vi "_Set BD Cluster Autosizing Property.vi"(8 "error in (no error)":errorcluster, 10 "type":T1(ring), 11 "SelList[]":refnum<vi>[](array[refnum])) -> (0 "error out":errorcluster, 3 "changed":bool)   [LabVIEW 2020, in "Cluster AutoSizing.lvlib"]
uses:
  Cluster AutoSizing.lvlib
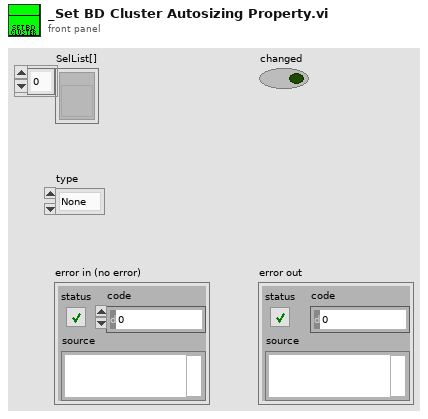
[diagram p1: front panel]
types:
  T1 = enum16{"None", "Size to Fit", "Arrange Horizontally", "Arrange Veritcally"}
  T2 = enum32{"None", "Size to Fit", "Arrange Horizontally", "Arrange Vertically"}
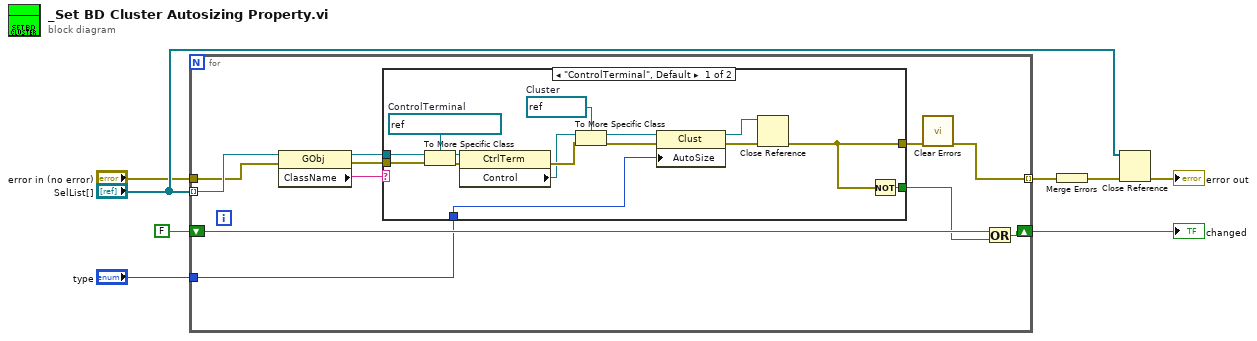
[diagram p0: block diagram]
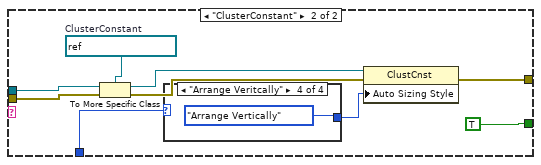
[diagram p2: hidden frame]
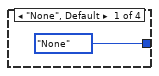
[diagram p3: hidden frame]
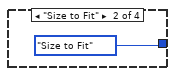
[diagram p4: hidden frame]
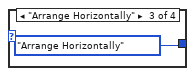
[diagram p5: hidden frame]
diagram:
  n1 = for {
    shift-right: [w18] -> w3
    shift-left: FALSE -> [w19]
    tunnel: "SelList[]" -> [w17] mode=indexing
    tunnel: "error in (no error)" -> [w12]
    tunnel: [w9] -> w4 mode=indexing
    tunnel: "type" -> [w16]
    n2 = property class="GObj"(reference=w17, error in=w12) -> (reference out=w14:refnum<vi>, error out=w13:errorcluster, "ClassName"=w11:string)
    n3 = case shown="\"ControlTerminal\", Default" w11 {
      tunnel: w16 -> [w20 w36]
      tunnel: [w21 w43] -> w15
      tunnel: w14 -> [w26 w42]
      tunnel: w13 -> [w25 w41]
      tunnel: [w22 TRUE] -> w10
      frame "ControlTerminal", Default {
        w30 = refnum<vi> refnum  # Cluster
        w24 = refnum<vi> refnum  # ControlTerminal
        n4 = To More Specific Class(target class=w24, reference=w26, error in=w25) -> (specific class reference=w34:refnum<vi>, error out=w33:errorcluster)
        n5 = property class="CtrlTerm"(reference=w34, error in=w33) -> (error out=w29:errorcluster, "Control"=w23:refnum<vi>)  [unwired: 1 out]
        n6 = To More Specific Class(target class=w30, reference=w23, error in=w29) -> (specific class reference=w32:refnum<vi>, error out=w31:errorcluster)
        n7 = property class="Clust"(reference=w32, error in=w31, "AutoSize"=w20) -> (reference out=w27:refnum<vi>, error out=w28:errorcluster)
        n8 = Close Reference(reference=w27, error in (no error)=w28) -> (error out=w21:errorcluster)
        n9 = Not(x=w21) -> (.not. x?=w22:bool)
      }
      frame "ClusterConstant" {
        w40 = refnum<vi> refnum  # ClusterConstant
        n10 = To More Specific Class(target class=w40, reference=w42, error in=w41) -> (specific class reference=w38:refnum<vi>, error out=w39:errorcluster)
        n11 = case shown="\"Arrange Veritcally\"" w36 {
          tunnel: [T2."None" ("Auto Sizing Style") T2."Size to Fit" ("Auto Sizing Style") T2."Arrange Horizontally" ("Auto Sizing Style") T2."Arrange Vertically" ("Auto Sizing Style")] -> w35
          frame "None", Default {
          }
          frame "Size to Fit" {
          }
          frame "Arrange Horizontally" {
          }
          frame "Arrange Veritcally" {
          }
        }
        n12 = property class="ClustCnst"(reference=w38, error in=w39, "Auto Sizing Style"=w35) -> (error out=w43:errorcluster)  [unwired: 1 out]
      }
    }
    n13 = call <vilib>:"Clear Errors.vi"("error in (no error)"=w15) -> ("error out"=w9:errorcluster)  [unwired: 5 in, 1 out]
    n14 = Or(x=w19, y=w10) -> (x .or. y?=w18:bool)
  }
  "changed" <- w3
  n15 = Merge Errors(w4) -> (w8:errorcluster)
  n16 = Close Reference(reference="SelList[]", error in (no error)=w8) -> (error out=→"error out":errorcluster)
